vi "FlushBufferToFile.vi"(8 "error in (no error)":errorcluster, 10 "tracepoints":T1[](array[typedef]), 11 "log dir":path) -> (0 "error out":errorcluster)   [LabVIEW 2017, in "TraceLogger.lvlib"]
uses:
  <vilib>/addons/TraceLogger/TraceLogger.lvlib
  <vilib>/addons/TraceLogger/controls/LogTracepoint.ctl
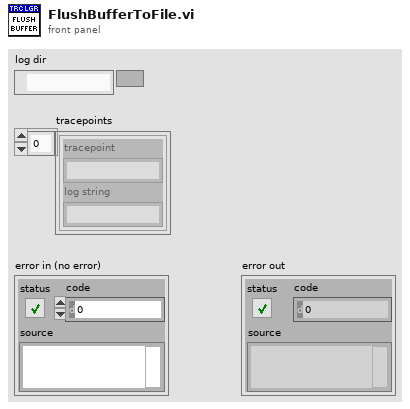
[diagram p1: front panel]
types:
  T1 = typedef "TraceLogger.lvlib/LogTracepoint.ctl" = cluster{"tracepoint":string, "log string":string}
  T2 = enum16{"open", "replace", "create", "open or create", "replace or create", "replace or create with confirmation"}
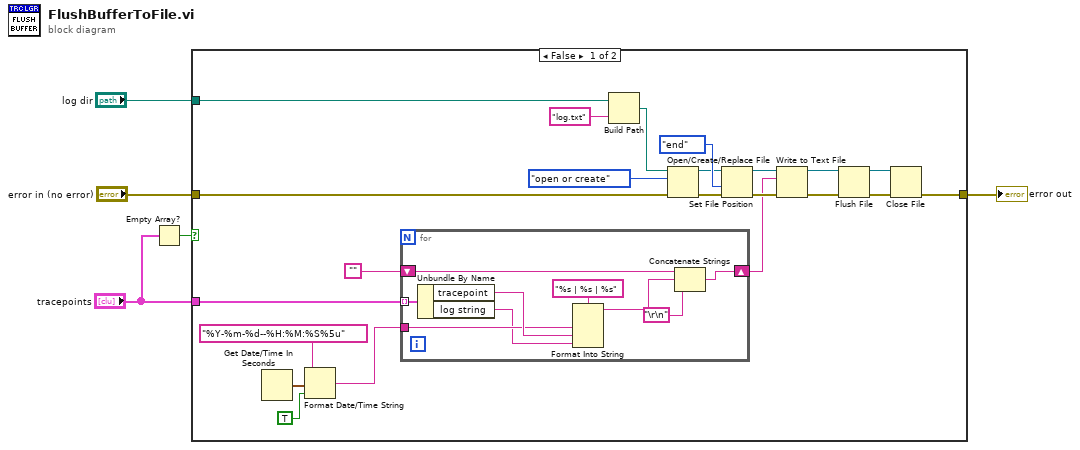
[diagram p0: block diagram]
diagram:
  n1 = Empty Array?(array="tracepoints") -> (empty?=w1:bool)
  n2 = case shown="False" w1 {
    tunnel: "log dir" -> [w21 _]
    tunnel: "error in (no error)" -> [w17 w37]
    tunnel: [w7 w37] -> w3
    tunnel: "tracepoints" -> [w11 _]
    frame False {
      n3 = Get Date/Time In Seconds() -> (seconds since 1Jan1904=w14:timestamp)
      n4 = Format Date/Time String(time format string (%c)="%Y-%m-%d--%H:%M:%S%5u", seconds (now)=w14, UTC format=TRUE) -> (date/time string=w12:string)
      n5 = for {
        shift-right: [w33] -> w16
        shift-left: "" -> [w35]
        tunnel: w11 -> [w36] mode=indexing
        tunnel: w12 -> [w30]
        n6 = Unbundle By Name(w36) -> ("tracepoint"=w31:string, "log string"=w29:string)
        n7 = Format Into String(format string="%s | %s | %s", w30, w31, w29) -> (resulting string=w28:string)  [unwired: 2 in, 1 out]
        n8 = Concatenate Strings(w35, w28, "\r\n") -> (w33:string)
      }
      n9 = Build Path(base path=w21, name or relative path="log.txt") -> (appended path=w19:path)
      n10 = Open/Create/Replace File(file path (use dialog)=w19, error in=w17, operation (0:open)=T2."open or create") -> (refnum out=w23:refnum<file>, error out=w24:errorcluster)  [unwired: 3 in, 1 out]
      n11 = Set File Position(refnum=w23, from (0:start)=enum16{"start", "end", "current"}."end", error in=w24) -> (refnum out=w26:refnum<file>, error out=w27:errorcluster)  [unwired: 1 in]
      n12 = Write to Text File(file (use dialog)=w26, text=w16, error in=w27) -> (refnum out=w8:refnum<file>, error out=w9:errorcluster)  [unwired: 1 in, 1 out]
      n13 = Flush File(refnum=w8, error in=w9) -> (refnum out=w6:refnum<file>, error out=w10:errorcluster)
      n14 = Close File(refnum=w6, error in=w10) -> (error out=w7:errorcluster)  [unwired: 1 out]
    }
    frame True {
    }
  }
  "error out" <- w3
